vi "Set Write Protect Code.vi"(7 "listen period":sgl=0.1, 8 "error in":errorcluster, 9 "Write Protect Code":u8(ring) items=["Not write protected", "Write protected", "Undefined"], 10 "Password":string="BROOKS  ", 11 "Brooks MFC in":refnum<class "Brooks MFC.lvclass">) -> (0 "error out":errorcluster, 2 "Write Protect Code":u8(ring) items=["Not write protected", "Write protected", "Undefined"], 3 "Brooks MFC out":refnum<class "Brooks MFC.lvclass">)   [LabVIEW 2016, in "Brooks MFC.lvclass"]
uses:
  Brooks MFC.lvclass
  Brooks MFC.lvclass/Brooks MFC.ctl
  Instance           3 30Saved   Set Write Protect Code .vi
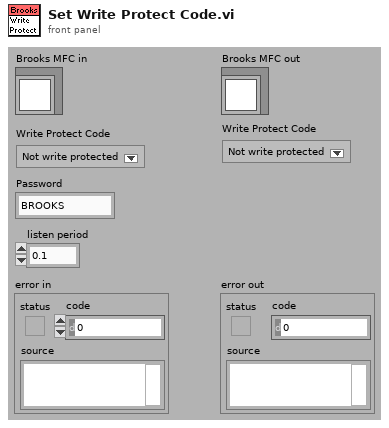
[diagram p1: front panel]
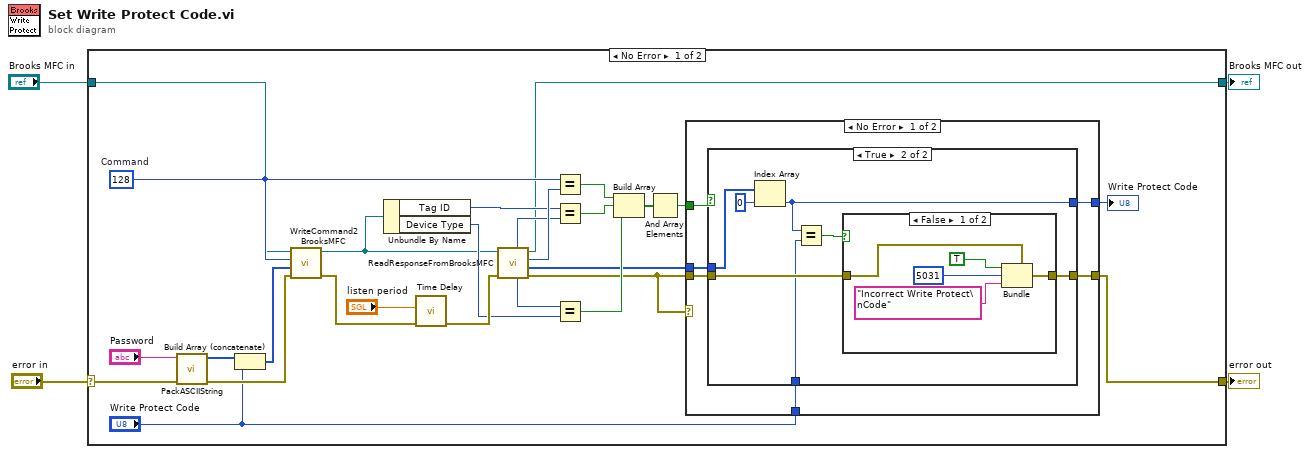
[diagram p0: block diagram]
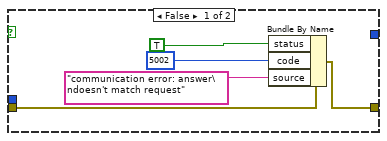
[diagram p2: hidden frame]
diagram:
  n1 = case shown="No Error" "error in" {
    selector: "error in" -> [w9 w58]
    tunnel: "Brooks MFC in" -> [w10 w57]
    tunnel: [w8 w58] -> w1
    tunnel: [w5 w57] -> w3
    frame No Error {
      w16 = u8 128  # Command
      n2 = call "PackASCIIString.vi"("Error In"=w9, "string"="Password") -> ("Error Out"=w19:errorcluster, "Packed Byte Array"=w18:u8[])  [unwired: 8 in]
      n3 = Build Array (concatenate)(w18, "Write Protect Code") -> (w15:u8[])
      n4 = call "WriteCommand2BrooksMFC.vi"("error in"=w19, "Data"=w15, "Command"=w16, "Brooks MFC in"=w10) -> ("error out"=w30:errorcluster, "Brooks MFC out"=w6:refnum<class "Brooks MFC.lvclass">)  [unwired: 5 in, 1 out]
      n5 = Unbundle By Name(w6) -> ("Tag ID"=w14:u32, "Device Type"=w13:u8)
      n6 = call "Time Delay"("error in (no error)"=w30, "Delay Time (s)"="listen period") -> ("error out"=w28:errorcluster)  [unwired: 9 in]
      n7 = call "ReadResponseFromBrooksMFC.vi"("error in"=w28, "Brooks MFC in"=w6) -> ("error out"=w11:errorcluster, "Data"=w7:u8[], "Command"=w31:u8, "Brooks MFC out"=w5:refnum<class "Brooks MFC.lvclass">, "device type"=w26:u8, "tag ID"=w27:u32)  [unwired: 4 in]
      n8 = Equal?(x=w16, y=w31) -> (x = y?=w25:bool)
      n9 = Equal?(x=w14, y=w27) -> (x = y?=w24:bool)
      n10 = Equal?(x=w26, y=w13) -> (x = y?=w23:bool)
      n11 = Build Array(w25, w24, w23) -> (w22:bool[])
      n12 = And Array Elements(Boolean array=w22) -> (logical AND=w21:bool)
      n13 = case shown="No Error" w11 {
        tunnel: w11 -> [w37 w56]
        tunnel: w7 -> [w36 _]
        tunnel: [w35 w56] -> w8
        tunnel: w21 -> [w34 _]
        tunnel: [w33 _] -> w17
        tunnel: "Write Protect Code" -> [w32 _]
        frame No Error {
          n14 = case shown="True" w34 {
            tunnel: w36 -> [_ w48]
            tunnel: w37 -> [w40 w46]
            tunnel: [w39 w47] -> w35
            tunnel: [_ w45] -> w33
            tunnel: w32 -> [_ w43]
            frame False {
              n15 = Bundle By Name(cluster=w40, "status"=TRUE ("Bundle Element"), "code"=5002 ("Bundle Element"), "source"="communication error: answer\ndoesn't match request") -> (w39:errorcluster)
            }
            frame True {
              n16 = Index Array(array=w48, index=0 ("Index")) -> (element=w45:u8)
              n17 = Equal?(x=w45, y=w43) -> (x = y?=w44:bool)
              n18 = case shown="False" w44 {
                tunnel: [w53 w55] -> w47
                tunnel: w46 -> [w54 w55]
                frame False {
                  n19 = Bundle(cluster=w54, "status"=TRUE, "code"=5031, "source"="Incorrect Write Protect\nCode") -> (w53:errorcluster)
                }
                frame True {
                }
              }
            }
          }
        }
        frame Error {
        }
      }
      "Write Protect Code" <- w17
    }
    frame Error {
    }
  }
  "Brooks MFC out" <- w3
  "error out" <- w1
